vi "demandsView.vi"(10 "UserEvents in":refnum<class "UserEvents.lvclass">) -> ()   [LabVIEW 2013]
uses:
  UserEvents/UserEvents.lvclass
  Typedefs/ForceDemand.ctl
  CommandFactory/CommandFactory.lvclass
  UserEvents/UserEvents.lvclass/UserEvents.ctl
  Typedefs/StateSelector.ctl
  Typedefs/CommandSelector.ctl
  Commands/StartAutomatedTest/StartAutomatedTest.lvclass
  Configuration/Test Parameters.ctl
  Configuration/CycleProfileConfig.ctl
  Commands/StartAutomatedTest/StartAutomatedTest.lvclass/StartAutomatedTest.ctl
  Commands/ForceDemand/ForceDemand.lvclass
  Commands/ForceDemand/ForceDemand.lvclass/ForceDemand.ctl
  Typedefs/M2AADTTypedefs.lvlib
  ConfigurationTestParameters/ConfigurationTestParameters.lvclass
panel:
  in  "enableMotionIsTrue":bool
  in  "sendForceDemandIsTrue":bool
  in  "stopMotionIsTrue":bool
  in  "stopAutomatedTestIsTrue":bool
  in  "startAutomatedTestIsTrue":bool
  in  "Force Demand":T1 format="%.6f"
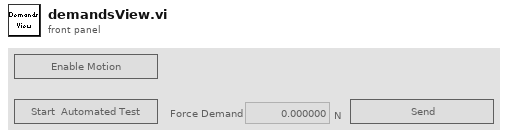
[diagram p1: front panel]
types:
  T1 = typedef "M2AADTTypedefs.lvlib/ForceDemand.ctl" = dbl[unit]
  T2 = enum8{"Enabled", "Disabled", "Disabled and Grayed Out"}
  T3 = typedef "M2AADTTypedefs.lvlib/PubDataEvents.ctl" = cluster{"State":refnum<user-event>, "ErrorCode":refnum<user-event>, "OutputData":refnum<user-event>, "InputData":refnum<user-event>, "ControllerData":refnum<user-event>, "TestStatus":refnum<user-event>, "LogPath":refnum<user-event>}
  T4 = typedef "M2AADTTypedefs.lvlib/SubDataEvents.ctl" = cluster{"Command":refnum<user-event>}
  T5 = cluster{"Event Registration Refnum":refnum<event-registration>}
  T6 = typedef "M2AADTTypedefs.lvlib/StateSelector.ctl" = enum16{"EndingCycleState", "FaultState", "InteractiveMotionState", "MovingToNewForceState", "OffState", "PausingState", "StandbyState", "StoppedState"}
  T7 = typedef "Test Parameters.ctl" = cluster{"Number of cycles for complete test":u32, "Cycle profile":T8, "Log Directory":path, "Max records per file":u32, "Comment":string}
  T8 = typedef "CycleProfileConfig.ctl" = cluster{"Force Setpoint":dbl[unit][], "Pause After":dbl[unit][]}
  T9 = typedef "M2AADTTypedefs.lvlib/CommandSelector.ctl" = enum16{"ClearError", "EnableMotion", "Exit", "ForceDemand", "StandBy", "Start", "StartAutomatedTest", "StopAutomatedTest", "StopMotion", "Update"}
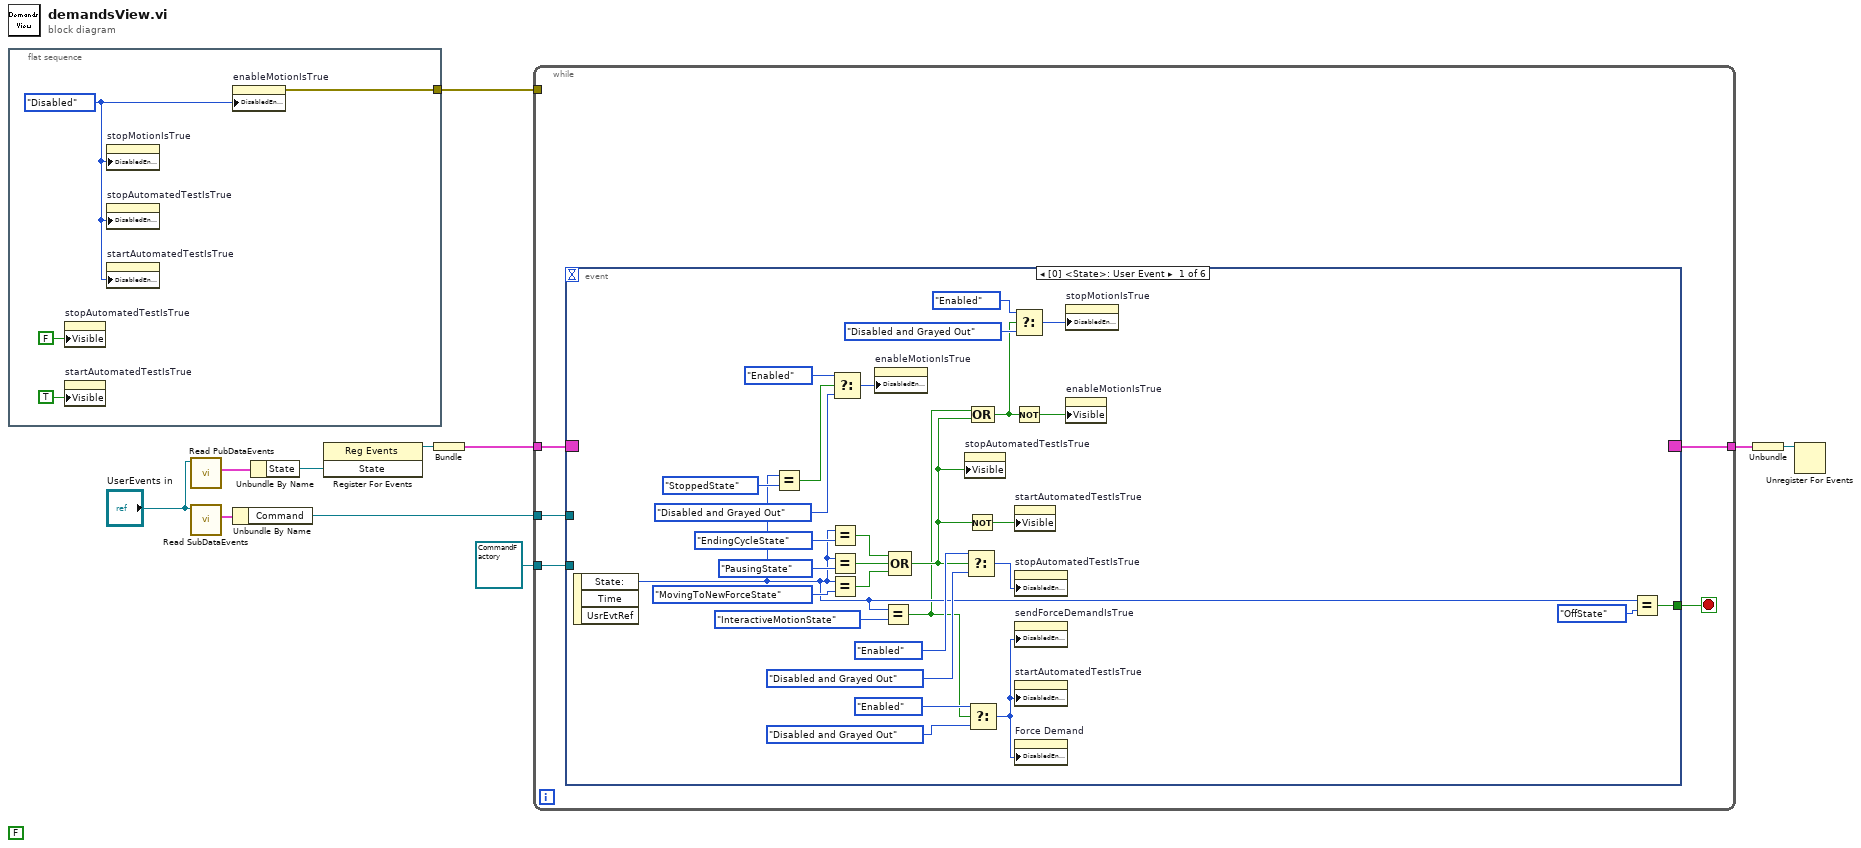
[diagram p0: block diagram]
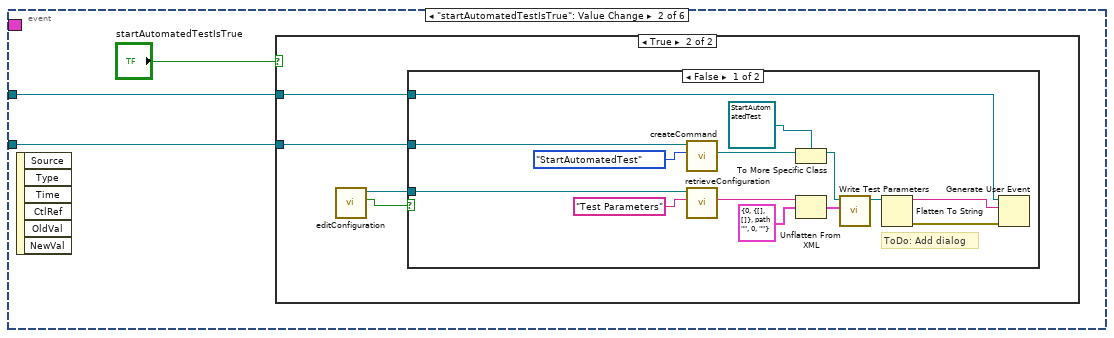
[diagram p2: hidden frame]
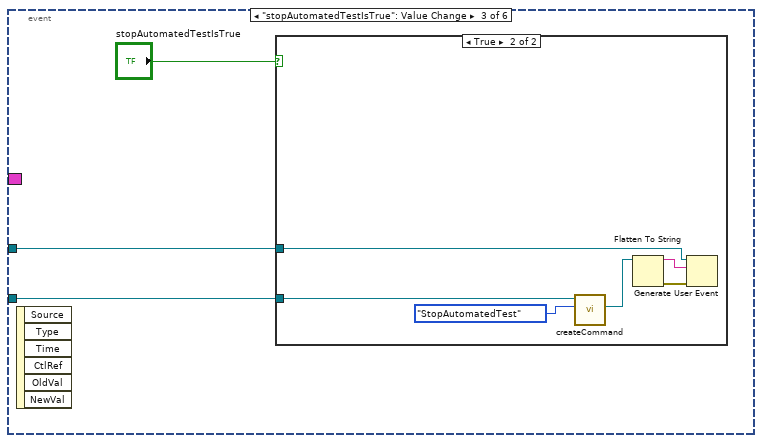
[diagram p5: hidden frame]
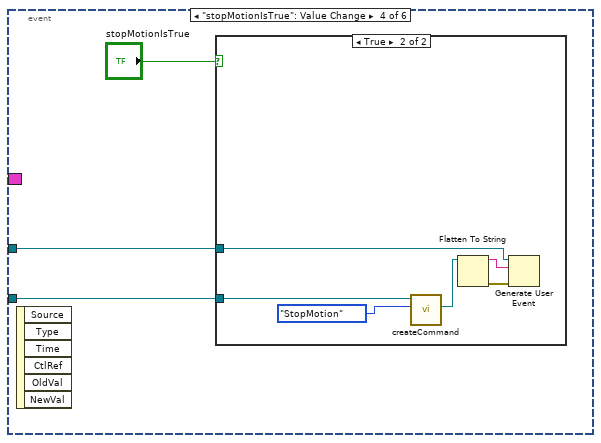
[diagram p7: hidden frame]
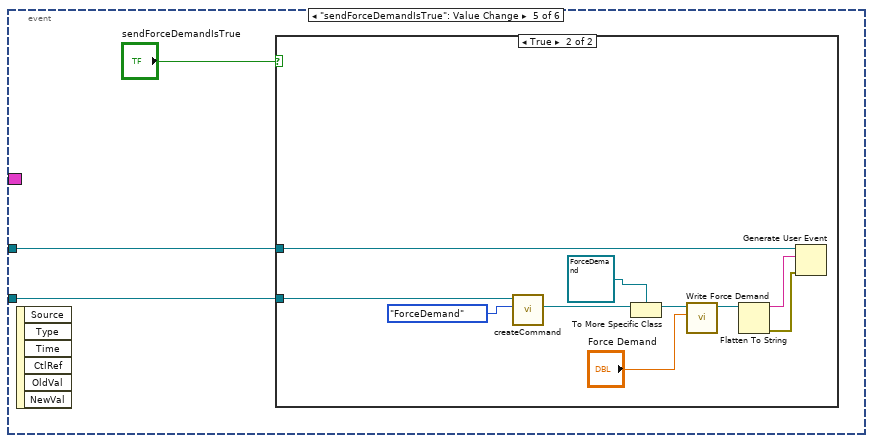
[diagram p9: hidden frame]
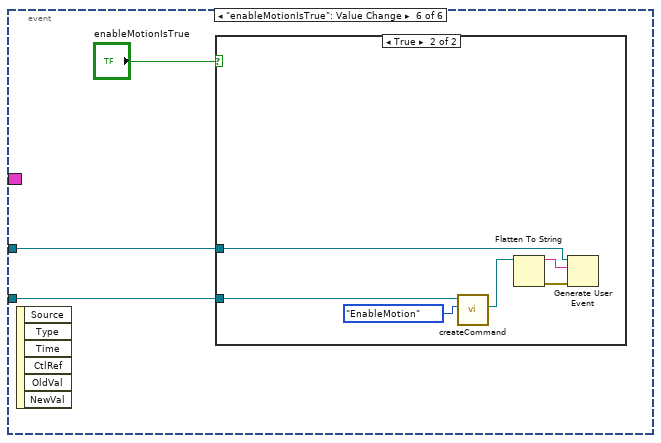
[diagram p11: hidden frame]
diagram:
  (unwired) FALSE ("motionInProgress")
  n1 = flat-sequence {
    tunnel: [w12] -> w1
    frame #0 {
      w15 = T2."Disabled" ("Disabled")
      n2 = property on="stopAutomatedTestIsTrue" class="Bool"("Visible"=FALSE) -> ()  [unwired: 2 in, 2 out]
      n3 = property on="startAutomatedTestIsTrue" class="Bool"("Visible"=TRUE) -> ()  [unwired: 2 in, 2 out]
      n4 = property on="stopMotionIsTrue" class="Bool"("DisabledEnum"=w15) -> ()  [unwired: 2 in, 2 out]
      n5 = property on="stopAutomatedTestIsTrue" class="Bool"("DisabledEnum"=w15) -> ()  [unwired: 2 in, 2 out]
      n6 = property on="startAutomatedTestIsTrue" class="Bool"("DisabledEnum"=w15) -> ()  [unwired: 2 in, 2 out]
      n7 = property on="enableMotionIsTrue" class="Bool"("DisabledEnum"=w15) -> (error out=w12:errorcluster)  [unwired: 2 in, 1 out]
    }
  }
  n8 = call "Read PubDataEvents.vi"("UserEvents in"="UserEvents in") -> ("PubDataEvents"=w8:T3)  [unwired: 9 in, 1 out]
  n9 = call "Read SubDataEvents.vi"("UserEvents in"="UserEvents in") -> ("SubDataEvents"=w9:T4)  [unwired: 9 in, 1 out]
  n10 = Unbundle By Name(w9) -> ("Command"=w6:refnum<user-event>)
  n11 = Unbundle By Name(w8) -> ("State"=w10:refnum<user-event>)
  n12 = register-events(w10) -> (reference out=w11:refnum<event-registration>)  [unwired: 2 in, 1 out]
  n13 = Bundle("Event Registration Refnum"=w11) -> (w7:T5)  [unwired: 1 in]
  n14 = while {
    tunnel: w7 -> [w20]
    tunnel: w6 -> [w19]
    tunnel: [w18] -> w5
    tunnel: refnum<class "CommandFactory.lvclass"> refnum ("CommandFactory.lvclass") -> [w16]
    tunnel: w1 -> [_]
    stop <- w17 stop-if-true
    n15 = event shown="[0] <State>: User Event" {
      selector: w20 -> [_ _ _ _ _ _]
      dyn-events: [_ _ _ _ _ _] -> w18
      timeout: _ -> [_ _ _ _ _ _]
      tunnel: w19 -> [_ w50 w73 w81 w91 w104]
      tunnel: [w46 _ _ _ _ _] -> w17
      tunnel: w16 -> [_ w51 w72 w80 w90 w103]
      event User Event {
        n16 = event-data() -> ("State:"=w26:T6)  [unwired: 1 in, 2 out]
        n17 = Equal?(x=w26, y=StateSelector."StoppedState") -> (x = y?=w23:bool)
        n18 = Equal?(x=w26, y=StateSelector."EndingCycleState") -> (x = y?=w37:bool)
        n19 = Equal?(x=w26, y=StateSelector."PausingState") -> (x = y?=w36:bool)
        n20 = Equal?(x=w26, y=StateSelector."MovingToNewForceState") -> (x = y?=w35:bool)
        n21 = Select(t=T2."Enabled" ("Disabled"), s=w23, f=T2."Disabled and Grayed Out" ("Disabled")) -> (s? t:f=w45:T2)
        n22 = property on="enableMotionIsTrue" class="Bool"("DisabledEnum"=w45) -> ()  [unwired: 2 in, 2 out]
        n23 = Equal?(x=w26, y=StateSelector."InteractiveMotionState") -> (x = y?=w25:bool)
        n24 = Compound Arithmetic op=OR(w37, w36, w35) -> (w30:bool)
        n25 = property on="stopAutomatedTestIsTrue" class="Bool"("Visible"=w30) -> ()  [unwired: 2 in, 2 out]
        n26 = Select(t=T2."Enabled" ("Disabled"), s=w30, f=T2."Disabled and Grayed Out" ("Disabled")) -> (s? t:f=w33:T2)
        n27 = Not(x=w30) -> (.not. x?=w31:bool)
        n28 = Select(t=T2."Enabled" ("Disabled"), s=w25, f=T2."Disabled and Grayed Out" ("Disabled")) -> (s? t:f=w24:T2)
        n29 = Compound Arithmetic op=OR(w25, w30) -> (w21:bool)
        n30 = Select(t=T2."Enabled" ("Disabled"), s=w21, f=T2."Disabled and Grayed Out" ("Disabled")) -> (s? t:f=w28:T2)
        n31 = Not(x=w21) -> (.not. x?=w22:bool)
        n32 = property on="startAutomatedTestIsTrue" class="Bool"("Visible"=w31) -> ()  [unwired: 2 in, 2 out]
        n33 = property on="stopAutomatedTestIsTrue" class="Bool"("DisabledEnum"=w33) -> ()  [unwired: 2 in, 2 out]
        n34 = property on="sendForceDemandIsTrue" class="Bool"("DisabledEnum"=w24) -> ()  [unwired: 2 in, 2 out]
        n35 = property on="startAutomatedTestIsTrue" class="Bool"("DisabledEnum"=w24) -> ()  [unwired: 2 in, 2 out]
        n36 = property on="Force Demand" class="DigNum (strict)"("DisabledEnum"=w24) -> ()  [unwired: 2 in, 2 out]
        n37 = property on="stopMotionIsTrue" class="Bool"("DisabledEnum"=w28) -> ()  [unwired: 2 in, 2 out]
        n38 = property on="enableMotionIsTrue" class="Bool"("Visible"=w22) -> ()  [unwired: 2 in, 2 out]
        n39 = Equal?(x=w26, y=StateSelector."OffState") -> (x = y?=w46:bool)
      }
      event "startAutomatedTestIsTrue": Value Change {
        n40 = event-data() -> ()  [unwired: 1 in, 6 out]
        n41 = case shown="True" "startAutomatedTestIsTrue" {
          tunnel: w51 -> [_ w56]
          tunnel: w50 -> [_ w55]
          frame False {
          }
          frame True {
            n42 = call "editConfiguration.vi"() -> ("cancelIsTrue out"=w53:bool, "ConfigurationThisComponent out"=w54:refnum<class "ConfigurationTestParameters.lvclass">)  [unwired: 9 in, 1 out]
            n43 = case shown="False" w53 {
              tunnel: w56 -> [w70 _]
              tunnel: w55 -> [w66 _]
              tunnel: w54 -> [w61 _]
              frame False {
                # "ToDo: Add dialog"
                n44 = call-dynamic "createCommand.vi"("Command"=CommandSelector."StartAutomatedTest", "CommandFactory in"=w70) -> ("command"=w65:refnum<class "Command.lvclass">)  [unwired: 7 in, 2 out]
                n45 = call "retrieveConfiguration.vi"("configName"="Test Parameters", "ConfigurationThisComponent in"=w61) -> ("xmlConfig"=w59:string)  [unwired: 7 in, 2 out]
                n46 = To More Specific Class(target class=refnum<class "StartAutomatedTest.lvclass"> refnum ("StartAutomatedTest.lvclass"), reference=w65) -> (specific class reference=w63:refnum<class "StartAutomatedTest.lvclass">)  [unwired: 1 in, 1 out]
                n47 = Unflatten From XML(xml string=w59, type=T7 {"Number of cycles for complete test"=0, "Cycle profile"={"Force Setpoint"=[], "Pause After"=[]}, "Log Directory"=path "", "Max records per file"=0, "Comment"=""} ("Test Parameters")) -> (value=w57:T7)  [unwired: 1 in, 1 out]
                n48 = call "Write Test Parameters.vi"("Test Parameters"=w57, "StartAutomatedTest in"=w63) -> ("StartAutomatedTest out"=w62:refnum<class "StartAutomatedTest.lvclass">)  [unwired: 9 in]
                n49 = Flatten To String(anything=w62) -> (data string=w67:string, error out=w68:errorcluster)  [unwired: 3 in, 1 out]
                n50 = Generate User Event(user event=w66, event data cluster=w67, error in=w68) -> ()  [unwired: 1 in, 2 out]
              }
              frame True {
              }
            }
          }
        }
      }
      event "stopAutomatedTestIsTrue": Value Change {
        n51 = event-data() -> ()  [unwired: 1 in, 6 out]
        n52 = case shown="True" "stopAutomatedTestIsTrue" {
          tunnel: w72 -> [_ w79]
          tunnel: w73 -> [_ w75]
          frame False {
          }
          frame True {
            n53 = call-dynamic "createCommand.vi"("Command"=CommandSelector."StopAutomatedTest", "CommandFactory in"=w79) -> ("command"=w74:refnum<class "Command.lvclass">)  [unwired: 7 in, 2 out]
            n54 = Flatten To String(anything=w74) -> (data string=w76:string, error out=w77:errorcluster)  [unwired: 3 in, 1 out]
            n55 = Generate User Event(user event=w75, event data cluster=w76, error in=w77) -> ()  [unwired: 1 in, 2 out]
          }
        }
      }
      event "stopMotionIsTrue": Value Change {
        n56 = event-data() -> ()  [unwired: 1 in, 6 out]
        n57 = case shown="True" "stopMotionIsTrue" {
          tunnel: w80 -> [_ w88]
          tunnel: w81 -> [_ w84]
          frame False {
          }
          frame True {
            n58 = call-dynamic "createCommand.vi"("Command"=CommandSelector."StopMotion", "CommandFactory in"=w88) -> ("command"=w83:refnum<class "Command.lvclass">)  [unwired: 7 in, 2 out]
            n59 = Flatten To String(anything=w83) -> (data string=w85:string, error out=w86:errorcluster)  [unwired: 3 in, 1 out]
            n60 = Generate User Event(user event=w84, event data cluster=w85, error in=w86) -> ()  [unwired: 1 in, 2 out]
          }
        }
      }
      event "sendForceDemandIsTrue": Value Change {
        n61 = event-data() -> ()  [unwired: 1 in, 6 out]
        n62 = case shown="True" "sendForceDemandIsTrue" {
          tunnel: w90 -> [_ w101]
          tunnel: w91 -> [_ w97]
          frame False {
          }
          frame True {
            n63 = call-dynamic "createCommand.vi"("Command"=CommandSelector."ForceDemand", "CommandFactory in"=w101) -> ("command"=w96:refnum<class "Command.lvclass">)  [unwired: 7 in, 2 out]
            n64 = To More Specific Class(target class=refnum<class "ForceDemand.lvclass"> refnum ("ForceDemand.lvclass"), reference=w96) -> (specific class reference=w94:refnum<class "ForceDemand.lvclass">)  [unwired: 1 in, 1 out]
            n65 = call "Write Force Demand.vi"("Force Demand"="Force Demand", "ForceDemand in"=w94) -> ("ForceDemand out"=w93:refnum<class "ForceDemand.lvclass">)  [unwired: 9 in]
            n66 = Flatten To String(anything=w93) -> (data string=w98:string, error out=w99:errorcluster)  [unwired: 3 in, 1 out]
            n67 = Generate User Event(user event=w97, event data cluster=w98, error in=w99) -> ()  [unwired: 1 in, 2 out]
          }
        }
      }
      event "enableMotionIsTrue": Value Change {
        n68 = event-data() -> ()  [unwired: 1 in, 6 out]
        n69 = case shown="True" "enableMotionIsTrue" {
          tunnel: w103 -> [_ w110]
          tunnel: w104 -> [_ w106]
          frame False {
          }
          frame True {
            n70 = call-dynamic "createCommand.vi"("Command"=CommandSelector."EnableMotion", "CommandFactory in"=w110) -> ("command"=w105:refnum<class "Command.lvclass">)  [unwired: 7 in, 2 out]
            n71 = Flatten To String(anything=w105) -> (data string=w107:string, error out=w108:errorcluster)  [unwired: 3 in, 1 out]
            n72 = Generate User Event(user event=w106, event data cluster=w107, error in=w108) -> ()  [unwired: 1 in, 2 out]
          }
        }
      }
    }
  }
  n73 = Unbundle(w5) -> ("Event Registration Refnum"=w4:refnum<event-registration>)
  n74 = Unregister For Events(event registration refnum=w4) -> ()  [unwired: 1 in, 1 out]
